vi "test_rethinkdb_json_performance.vi"(8 "error in (no error)":errorcluster) -> (0 "error out":errorcluster)   [LabVIEW 2017]
uses:
  <vilib>/Analysis/baseanly.llb/Mean (DBL).vi
  <vilib>/Analysis/NI_AALBase.lvlib
panel:
  out "element count":i32
  out "elements":T1(array[cluster])
  out "ms_min":dbl
  out "ms_max":dbl
  in  "iterations":i32=1000
  in  "json":string="[\n  {\n    \"_id\": \"5d4455b2c0f1933bd2d334b3\",\n    \"index\": 0,\n    \"guid\": \"2c98a9b2-612f-4acc-bb66-5b8509fb5632\",\n    \"isActive\": false,\n    \"balance\": \"$1,409.53\",\n    \"picture\": \"http://placehold.it/32x32\",\n    \"age\": 35,\n    \"eyeColor\": \"brown\",\n    \"name\": \"Tamera Douglas\",\n    \"gender\": \"female\",\n    \"company\": \"INSURON\",\n    \"email\": \"tameradouglas@insuron.com\",\n    \"phone\": \"+1 (946) 468-2681\",\n    \"address\": \"454 Oceanview Avenue, Axis, New Mexico, 4566\",\n    \"about\": \"Enim cillum cupidatat consectetur minim id consequat irure magna tempor deserunt. Reprehenderit Lorem enim deserunt eiusmod et excepteur in eiusmod ullamco sint minim exercitation laborum duis. Aute amet mollit tempor adipisicing. Eiusmod tempor qui proident amet sint eiusmod laborum nisi consectetur. Excepteur occaecat et consequat pariatur pariatur sit deserunt proident commodo enim sit do. Duis fugiat irure esse ipsum non nulla ut aliquip esse nisi. Mollit commodo sit elit amet duis nisi sint.\r\n\",\n    \"registered\": \"2019-04-15T12:36:48 +06:00\",\n    \"latitude\": 7.38495,\n    \"longitude\": -44.890348,\n    \"tags\": [\n      \"cillum\",\n      \"nisi\",\n      \"mollit\",\n      \"sunt\",\n      \"minim\",\n      \"non\",\n      \"ex\"\n    ],\n    \"friends\": [\n      {\n        \"id\": 0,\n        \"name\": \"Winnie Reid\"\n      },\n      {\n        \"id\": 1,\n        \"name\": \"Araceli Delacruz\"\n      },\n      {\n        \"id\": 2,\n        \"name\": \"Bolton Horne\"\n      }\n    ],\n    \"greeting\": \"Hello, Tamera Douglas! You have 1 unread messages.\",\n    \"favoriteFruit\": \"banana\"\n  },\n  {\n    \"_id\": \"5d4455b247ae2b298863909d\",\n    \"index\": 1,\n    \"guid\": \"00a03766-a5ca-45cc-8dfb-1ef19cade6a5\",\n    \"isActive\": true,\n    \"balance\": \"$2,933.39\",\n    \"picture\": \"http://placehold.it/32x32\",\n    \"age\": 30,\n    \"eyeColor\": \"blue\",\n    \"name\": \"Garner Hooper\",\n    \"gender\": \"male\",\n    \"company\": \"SENMEI\",\n    \"email\": \"garnerhooper@senmei.com\",\n    \"phone\": \"+1 (805) 444-2443\",\n    \"address\": \"334 Herkimer Place, Westphalia, West Virginia, 8777\",\n    \"about\": \"Tempor tempor commodo do cillum ex. Velit minim esse nulla incididunt cupidatat. Aliqua tempor magna pariatur incididunt nostrud id cupidatat aliquip elit est ullamco. Mollit magna ut deserunt nisi exercitation reprehenderit proident ipsum occaecat ut enim. Voluptate adipisicing culpa veniam duis amet.\r\n\",\n    \"registered\": \"2019-02-20T09:03:35 +07:00\",\n    \"latitude\": 3.634789,\n    \"longitude\": -71.711449,\n    \"tags\": [\n      \"laboris\",\n      \"sunt\",\n      \"elit\",\n      \"esse\",\n      \"aliqua\",\n      \"nulla\",\n      \"in\"\n    ],\n    \"friends\": [\n      {\n        \"id\": 0,\n        \"name\": \"Saundra Mullen\"\n      },\n      {\n        \"id\": 1,\n        \"name\": \"Macdonald Houston\"\n      },\n      {\n        \"id\": 2,\n        \"name\": \"Rivera Hyde\"\n      }\n    ],\n    \"greeting\": \"Hello, Garner Hooper! You have 1 unread messages.\",\n    \"favoriteFruit\": \"banana\"\n  },\n  {\n    \"_id\": \"5d4455b288b3a8bcda8c1081\",\n    \"index\": 2,\n    \"guid\": \"14e7d77e-1ed5-4b08-bdae-19e0328d29f8\",\n    \"isActive\": false,\n    \"balance\": \"$1,321.03\",\n    \"picture\": \"http://placehold.it/32x32\",\n    \"age\": 33,\n    \"eyeColor\": \"blue\",\n    \"name\": \"Neal Buckley\",\n    \"gender\": \"male\",\n    \"company\": \"TRIBALOG\",\n    \"email\": \"nealbuckley@tribalog.com\",\n    \"phone\": \"+1 (879) 521-3254\",\n    \"address\": \"378 Preston Court, Unionville, Northern Mariana Islands, 6583\",\n    \"about\": \"Elit enim consectetur ad non tempor ad tempor proident do. In consectetur fugiat commodo ex. Ut nulla voluptate aliquip esse. Officia esse proident minim enim cillum deserunt mollit. Anim do deserunt amet velit consequat anim ullamco enim Lorem esse culpa irure voluptate labore. Laboris officia officia aliqua elit elit non culpa cillum dolore amet quis.\r\n\",\n    \"registered\": \"2019-01-23T03:40:45 +07:00\",\n    \"latitude\": 8.381404,\n    \"longitude\": -96.636286,\n    \"tags\": [\n      \"velit\",\n      \"esse\",\n      \"id\",\n      \"ullamco\",\n      \"sunt\",\n      \"amet\",\n      \"ad\"\n    ],\n    \"friends\": [\n      {\n        \"id\": 0,\n        \"name\": \"Hall Booker\"\n      },\n      {\n        \"id\": 1,\n        \"name\": \"Lawson Stevenson\"\n      },\n      {\n        \"id\": 2,\n        \"name\": \"Maynard Gill\"\n      }\n    ],\n    \"greeting\": \"Hello, Neal Buckley! You have 9 unread messages.\",\n    \"favoriteFruit\": \"apple\"\n  },\n  {\n    \"_id\": \"5d4455b21a3db63bef3f777a\",\n    \"index\": 3,\n    \"guid\": \"d4ea16a6-f1ec-4bfe-9970-657798a14ac1\",\n    \"isActive\": false,\n    \"balance\": \"$2,499.94\",\n    \"picture\": \"http://placehold.it/32x32\",\n    \"age\": 37,\n    \"eyeColor\": \"green\",\n    \"name\": \"Marguerite Gay\",\n    \"gender\": \"female\",\n    \"company\": \"DADABASE\",\n    \"email\": \"margueritegay@dadabase.com\",\n    \"phone\": \"+1 (937) 434-3754\",\n    \"address\": \"256 Dooley Street, Sylvanite, Nevada, 1343\",\n    \"about\": \"Aute elit laborum cillum minim esse ex eu est. Cillum in esse irure ut do duis et eiusmod aliqua et adipisicing. Sunt adipisicing commodo dolor sit qui laborum commodo deserunt amet minim. Proident sint labore consequat commodo enim veniam veniam ea amet eu qui. Officia culpa dolor adipisicing laborum. Commodo elit sunt anim laboris laborum amet nulla.\r\n\",\n    \"registered\": \"2014-05-27T12:57:25 +06:00\",\n    \"latitude\": 64.083884,\n    \"longitude\": -30.078651,\n    \"tags\": [\n      \"minim\",\n      \"mollit\",\n      \"laboris\",\n      \"pariatur\",\n      \"qui\",\n      \"sit\",\n      \"do\"\n    ],\n    \"friends\": [\n      {\n        \"id\": 0,\n        \"name\": \"Duffy Steele\"\n      },\n      {\n        \"id\": 1,\n        \"name\": \"Preston Lamb\"\n      },\n      {\n        \"id\": 2,\n        \"name\": \"Velasquez Shaffer\"\n      }\n    ],\n    \"greeting\": \"Hello, Marguerite Gay! You have 5 unread messages.\",\n    \"favoriteFruit\": \"apple\"\n  },\n  {\n    \"_id\": \"5d4455b2664446faf7994a00\",\n    \"index\": 4,\n    \"guid\": \"75fe4cd8-2ec4-47e4-9a35-4a72f803cd01\",\n    \"isActive\": true,\n    \"balance\": \"$3,522.35\",\n    \"picture\": \"http://placehold.it/32x32\",\n    \"age\": 20,\n    \"eyeColor\": \"brown\",\n    \"name\": \"Graciela Orr\",\n    \"gender\": \"female\",\n    \"company\": \"ENTROFLEX\",\n    \"email\": \"gracielaorr@entroflex.com\",\n    \"phone\": \"+1 (855) 541-3462\",\n    \"address\": \"895 Sapphire Street, Ruckersville, Georgia, 6484\",\n    \"about\": \"Consectetur reprehenderit laboris minim anim aute aliquip Lorem ullamco non consequat. Tempor officia occaecat eu amet quis quis fugiat. Eu ad ex elit dolor. Do proident veniam aute irure consectetur laborum nulla qui Lorem ut culpa commodo. Quis commodo commodo sint sunt veniam. Magna commodo reprehenderit duis eu deserunt qui amet. Pariatur ut occaecat minim officia commodo voluptate esse in id anim.\r\n\",\n    \"registered\": \"2017-02-22T08:24:12 +07:00\",\n    \"latitude\": -84.018578,\n    \"longitude\": 66.386099,\n    \"tags\": [\n      \"excepteur\",\n      \"anim\",\n      \"commodo\",\n      \"amet\",\n      \"consequat\",\n      \"tempor\",\n      \"quis\"\n    ],\n    \"friends\": [\n      {\n        \"id\": 0,\n        \"name\": \"Ollie Cline\"\n      },\n      {\n        \"id\": 1,\n        \"name\": \"Corina Powers\"\n      },\n      {\n        \"id\": 2,\n        \"name\": \"Lynda Workman\"\n      }\n    ],\n    \"greeting\": \"Hello, Graciela Orr! You have 6 unread messages.\",\n    \"favoriteFruit\": \"apple\"\n  },\n  {\n    \"_id\": \"5d4455b2ca59b0a7fc9c71cd\",\n    \"index\": 5,\n    \"guid\": \"a5d705b7-9c22-4a73-968c-37b6847d31de\",\n    \"isActive\": true,\n    \"balance\": \"$2,719.98\",\n    \"picture\": \"http://placehold.it/32x32\",\n    \"age\": 30,\n    \"eyeColor\": \"blue\",\n    \"name\": \"Lynn Durham\",\n    \"gender\": \"male\",\n    \"company\": \"RODEOMAD\",\n    \"email\": \"lynndurham@rodeomad.com\",\n    \"phone\": \"+1 (896) 522-2325\",\n    \"address\": \"202 Erskine Loop, Silkworth, North Dakota, 8325\",\n    \"about\": \"Anim sunt irure ut sint. Ullamco consectetur non pariatur consectetur ullamco. Consequat cupidatat nisi eiusmod magna ut eiusmod. Ullamco cillum culpa voluptate fugiat laboris nulla Lorem ad irure ipsum mollit.\r\n\",\n    \"registered\": \"2017-06-19T08:42:14 +06:00\",\n    \"latitude\": -19.936145,\n    \"longitude\": 149.259571,\n    \"tags\": [\n      \"ea\",\n      \"proident\",\n      \"tempor\",\n      \"cillum\",\n      \"sit\",\n      \"veniam\",\n      \"velit\"\n    ],\n    \"friends\": [\n      {\n        \"id\": 0,\n        \"name\": \"Horne Kelley\"\n      },\n      {\n        \"id\": 1,\n        \"name\": \"Elvia Harper\"\n      },\n      {\n        \"id\": 2,\n        \"name\": \"Hooper Griffith\"\n      }\n    ],\n    \"greeting\": \"Hello, Lynn Durham! You have 2 unread messages.\",\n    \"favoriteFruit\": \"banana\"\n  },\n  {\n    \"_id\": \"5d4455b2293b6080ad5e354a\",\n    \"index\": 6,\n    \"guid\": \"64e7c98c-aecf-4ff2-aeff-e95c9629e4fa\",\n    \"isActive\": false,\n    \"balance\": \"$3,702.37\",\n    \"picture\": \"http://placehold.it/32x32\",\n    \"age\": 22,\n    \"eyeColor\": \"brown\",\n    \"name\": \"Bethany Salazar\",\n    \"gender\": \"female\",\n    \"company\": \"TRIPSCH\",\n    \"email\": \"bethanysalazar@tripsch.com\",\n    \"phone\": \"+1 (856) 524-3649\",\n    \"address\": \"754 Prospect Place, Crumpler, Palau, 1899\",\n    \"about\": \"Tempor non occaecat veniam non. Mollit exercitation magna eiusmod cillum. Consequat do irure deserunt velit. Consectetur aute deserunt esse anim nostrud do.\r\n\",\n    \"registered\": \"2014-09-10T09:21:42 +06:00\",\n    \"latitude\": -55.3388,\n    \"longitude\": -63.497523,\n    \"tags\": [\n      \"incididunt\",\n      \"cupidatat\",\n      \"voluptate\",\n      \"pariatur\",\n      \"dolore\",\n      \"tempor\",\n      \"laborum\"\n    ],\n    \"friends\": [\n      {\n        \"id\": 0,\n        \"name\": \"Weiss Hahn\"\n      },\n      {\n        \"id\": 1,\n        \"name\": \"Trudy Roy\"\n      },\n      {\n        \"id\": 2,\n        \"name\": \"Schultz Vazquez\"\n      }\n    ],\n    \"greeting\": \"Hello, Bethany Salazar! You have 4 unread messages.\",\n    \"favoriteFruit\": \"banana\"\n  }\n]"
  out "ms_avg":dbl
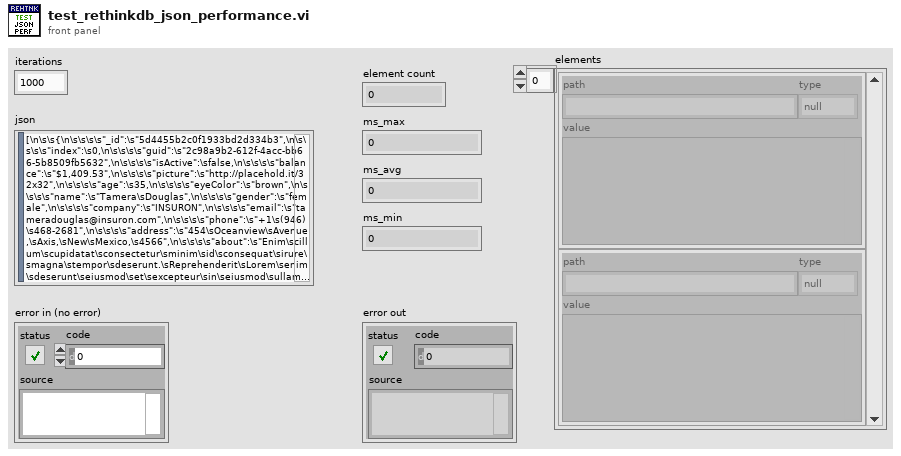
[diagram p1: front panel]
types:
  T1 = cluster{"path":string, "type":enum8{"null", "bool", "int", "uint", "float", "string", "array", "object"}, "value":variant}[]
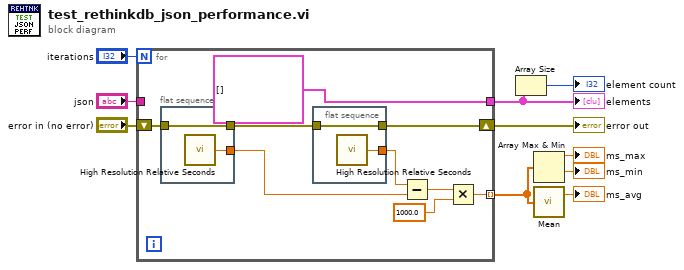
[diagram p0: block diagram]
diagram:
  n1 = for {
    N: "iterations" -> [_]
    tunnel: [w17] -> w4 mode=indexing
    tunnel: "json" -> [_]
    tunnel: [T1 [] ("elements")] -> w2
    shift-right: [w18] -> w9
    shift-left: "error in (no error)" -> [w19]
    n2 = flat-sequence {
      tunnel: [w23] -> w11
      tunnel: w19 -> [w23]
      tunnel: [w22] -> w15
      frame #0 {
        n3 = call <vilib>:"High Resolution Relative Seconds.vi"() -> ("relative seconds"=w22:dbl)
      }
    }
    n4 = flat-sequence {
      tunnel: [w21] -> w18
      tunnel: w11 -> [w21]
      tunnel: [w20] -> w16
      frame #0 {
        n5 = call <vilib>:"High Resolution Relative Seconds.vi"() -> ("relative seconds"=w20:dbl)
      }
    }
    n6 = Subtract(x=w16, y=w15) -> (x-y=w14:dbl)
    n7 = Multiply(x=w14, y=1000.0) -> (x*y=w17:dbl)
  }
  "error out" <- w9
  "elements" <- w2
  n8 = Array Size(array=w2) -> (size(s)=→"element count":i32)
  n9 = Array Max & Min(array=w4) -> (max value=→"ms_max":dbl, min value=→"ms_min":dbl)  [unwired: 2 out]
  n10 = call-poly <vilib>:"Mean.vi"("X"=w4) -> ("mean"=→"ms_avg":dbl)  [unwired: 1 out]
